vi "AdvServoCount.vi"(8 "error in (no error)":errorcluster, 11 "Device In":i32) -> (0 "error out":errorcluster, 2 "count":i32, 3 "Device Out":i32)   [LabVIEW 2014]
uses:
  phidget21.dll
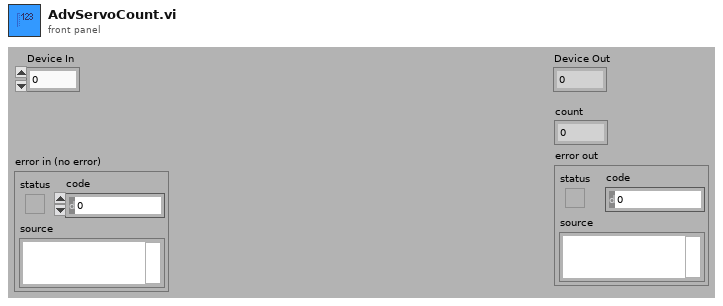
[diagram p1: front panel]
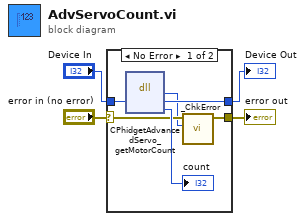
[diagram p0: block diagram]
diagram:
  n1 = case shown="No Error" "error in (no error)" {
    selector: "error in (no error)" -> [w7 w12]
    tunnel: [w6 w12] -> w3
    tunnel: "Device In" -> [w9 w11]
    tunnel: [w8 w11] -> w1
    frame No Error {
      n2 = dll-call lib="phidget21.*" fn="CPhidgetAdvancedServo_getMotorCount"("phid"=w9) -> (w5:i32, "phid"=w8:i32, "count"=→"count":i32)  [unwired: 4 in, 2 out]
      n3 = call "_ChkError.vi"("Return Code"=w5, "error in (no error)"=w7) -> ("error out"=w6:errorcluster)  [unwired: 9 in]
    }
    frame Error {
    }
  }
  "error out" <- w3
  "Device Out" <- w1
